vi "getStartStopReleaseTime.vi"(10 "Control Parameter":T1, 11 "Day Time":u32) -> (3 "Activity (on / off)":i64)   [LabVIEW 2017]
panel:
  out "Stop Time":dbl
  out "Start Time":dbl
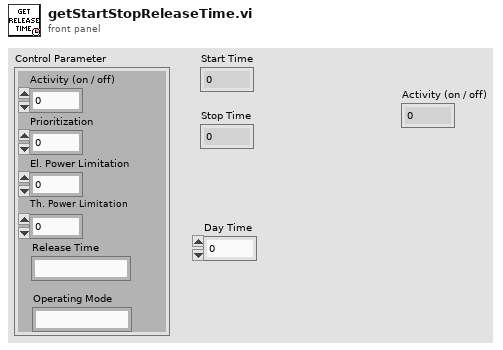
[diagram p1: front panel]
types:
  T1 = cluster{"Activity (on / off)":i64, "Prioritization":i64, "El. Power Limitation":dbl, "Th. Power Limitation":dbl, "Release Time":string, "Operating Mode":string}
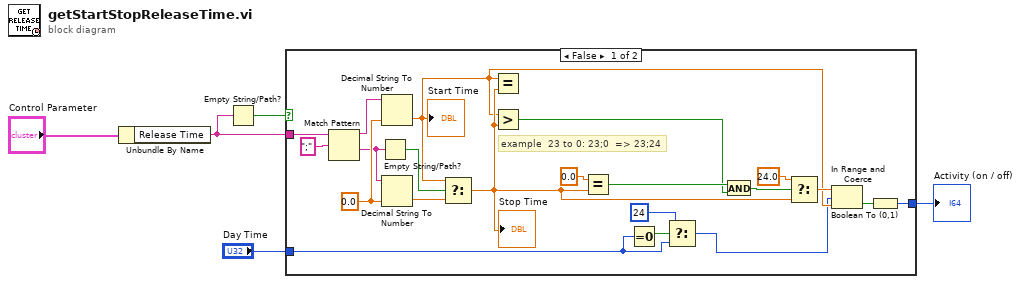
[diagram p0: block diagram]
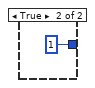
[diagram p2: hidden frame]
diagram:
  n1 = Unbundle By Name("Control Parameter") -> ("Release Time"=w2:string)
  n2 = Empty String/Path?(string/path=w2) -> (empty?=w1:bool)
  n3 = case shown="False" w1 {
    tunnel: [w22 i16 1] -> w4
    tunnel: "Day Time" -> [w8 _]
    tunnel: w2 -> [w15 _]
    frame False {
      w26 = 0.0 ("Power Out")
      # "example  23 to 0: 23;0  => 23;24"
      n4 = Match Pattern(string=w15, regular expression=";") -> (before substring=w25:string, after substring=w14:string)  [unwired: 1 in, 2 out]
      n5 = Empty String/Path?(string/path=w14) -> (empty?=w12:bool)
      n6 = Decimal String To Number(string=w25, default (0L)=w26) -> (number=w10:dbl)  [unwired: 1 in, 1 out]
      "Start Time" <- w10
      n7 = Decimal String To Number(string=w14, default (0L)=w26) -> (number=w13:dbl)  [unwired: 1 in, 1 out]
      n8 = Select(t=w10, s=w12, f=w13) -> (s? t:f=w11:dbl)
      "Stop Time" <- w11
      n9 = Equal?(x=w10, y=w11) -> ()  [unwired: 1 out]
      n10 = Greater?(x=w10, y=w11) -> (0:w19:bool)
      n11 = Equal?(x=0.0, y=w11) -> (x = y?=w20:bool)
      n12 = Equal To 0?(x=w8) -> (x = 0?=w9:bool)
      n13 = Select(t=u32 24, s=w9, f=w8) -> (s? t:f=w7:u32)
      n14 = And(x=w20, y=w19) -> (x .and. y?=w18:bool)
      n15 = Select(t=24.0, s=w18, f=w11) -> (s? t:f=w16:dbl)
      n16 = In Range and Coerce(upper limit=w16, x=w7, lower limit=w10) -> (In Range?=w23:bool)  [unwired: 1 out]
      n17 = Boolean To (0,1)(Boolean=w23) -> (0, 1=w22:i16)
    }
    frame True {
    }
  }
  "Activity (on / off)" <- w4
